vi "Read Y_Source.vi"(8 "error in (no error)":errorcluster, 11 "Y_H in":refnum<class "Y_H.lvclass">) -> (0 "error out":errorcluster, 2 "Y_Source":T1, 3 "Y_H out":refnum<class "Y_H.lvclass">)   [LabVIEW 2019, in "Y_H.lvclass"]
uses:
  Y_H.lvclass
  Reg/ctl/Y_source.ctl
  Y_H.lvclass/Y_H.ctl
  Reg/control.lvlib
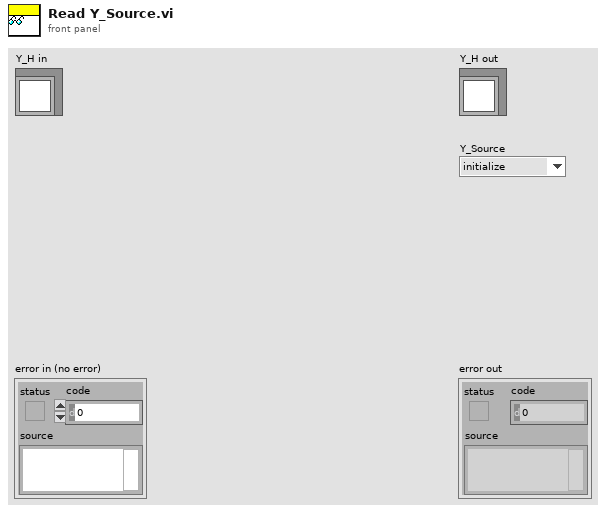
[diagram p1: front panel]
types:
  T1 = typedef "control.lvlib/Y_source.ctl" = enum8{"initialize", "local disabled", "local hand", "hand", "auto", "dist"}
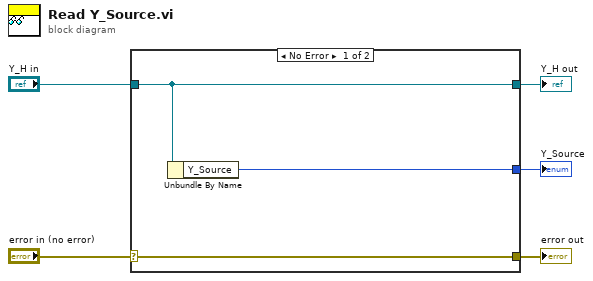
[diagram p0: block diagram]
diagram:
  n1 = case shown="No Error" "error in (no error)" {
    selector: "error in (no error)" -> [w8 w9]
    tunnel: [w8 w9] -> w4
    tunnel: [w7 w10] -> w2
    tunnel: "Y_H in" -> [w7 w10]
    tunnel: [w6 _] -> w1
    frame No Error {
      n2 = Unbundle By Name(w7) -> ("Y_Source"=w6:T1)
    }
    frame Error {
    }
  }
  "error out" <- w4
  "Y_H out" <- w2
  "Y_Source" <- w1
